vi "SetOutputMode.vi"(8 "error in (no error)":errorcluster, 10 "totempole":bool, 11 "PCA in":refnum<class "PCA.lvclass">) -> (0 "error out":errorcluster, 3 "PCA out":refnum<class "PCA.lvclass">)   [LabVIEW 2022 SP3, in "PCA9685.lvlib" / "PCA.lvclass"]
uses:
  PCA.lvclass
  PCA.lvclass/PCA.ctl
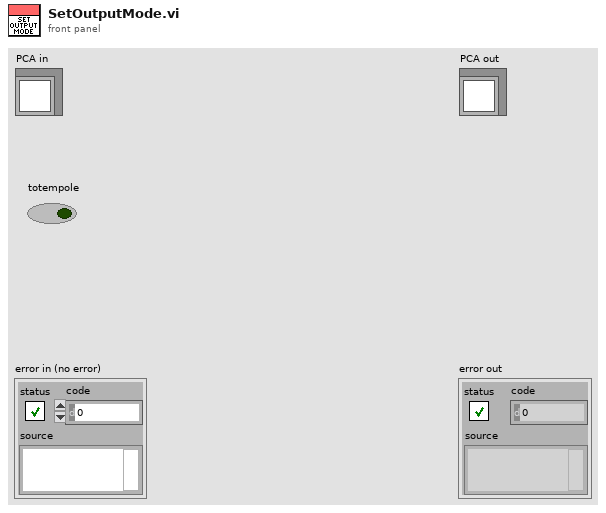
[diagram p1: front panel]
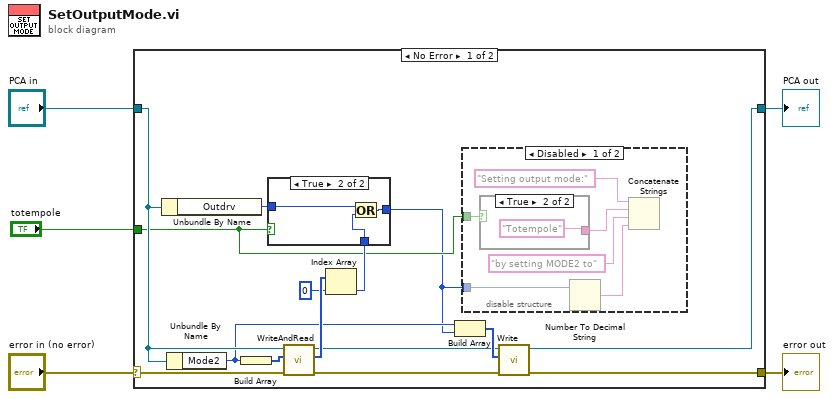
[diagram p0: block diagram]
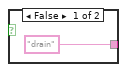
[diagram p2: hidden frame]
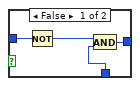
[diagram p4: hidden frame]
diagram:
  n1 = case shown="No Error" "error in (no error)" {
    selector: "error in (no error)" -> [w20 w37]
    tunnel: [w15 w37] -> w4
    tunnel: [w8 w36] -> w2
    tunnel: "PCA in" -> [w18 w36]
    tunnel: "totempole" -> [w7 _]
    frame No Error {
      n2 = Unbundle By Name(w18) -> ("Outdrv"=w17:u8)
      n3 = Unbundle By Name(w18) -> ("Mode2"=w11:u8)
      n4 = Build Array(w11) -> (w19:u8[])
      n5 = call "WriteAndRead.vi"("error in (no error)"=w20, "Data"=w19, "PCA in"=w18) -> ("error out"=w16:errorcluster, "Data 2"=w14:u8[], "PCA out"=w9:refnum<class "PCA.lvclass">)  [unwired: 6 in]
      n6 = Index Array(array=w14, index=0) -> (element=w12:u8)
      n7 = case shown="True" w7 {
        tunnel: w17 -> [w32 w34]
        tunnel: w12 -> [w31 w35]
        tunnel: [w29 w33] -> w6
        frame False {
          n8 = Not(x=w32) -> (.not. x?=w30:u8)
          n9 = And(x=w30, y=w31) -> (x .and. y?=w29:u8)
        }
        frame True {
          n10 = Or(x=w34, y=w35) -> (x .or. y?=w33:u8)
        }
      }
      n11 = Build Array(w11, w6) -> (w10:u8[])
      n12 = disable-structure shown="Disabled" {
        disable-tunnel: w7 -> [w25 _]
        disable-tunnel: w6 -> [w22 _]
        frame Disabled {
          n13 = case shown="True" w25 {
            tunnel: ["drain" "Totempole"] -> w24
            frame False {
            }
            frame True {
            }
          }
          n14 = Number To Decimal String(number=w22) -> (decimal integer string=w21:string)  [unwired: 1 in]
          n15 = Concatenate Strings("Setting output mode:" ("format string"), w24, "by setting MODE2 to" ("string"), w21) -> ()  [unwired: 1 out]
        }
        frame Enabled {
        }
      }
      n16 = call "Write.vi"("error in (no error)"=w16, "Data"=w10, "PCA in"=w9) -> ("error out"=w15:errorcluster, "PCA out"=w8:refnum<class "PCA.lvclass">)  [unwired: 7 in]
    }
    frame Error {
    }
  }
  "error out" <- w4
  "PCA out" <- w2
